vi "视频播放.vi"() -> ()   [LabVIEW 2014]
panel:
  out "Image 2":T1(plugin-control)
  out "Image":T1(plugin-control)
  in  "Image Type":T2 items=["Grayscale (U8)", "Grayscale (I16)", "Grayscale (SGL)", "Complex (CSG)", "RGB (U32)", "HSL (U32)", "RGB (U64)", "Grayscale (U16)"]
  in  "Image Name":string="untitled"
  in  "AVI Path":path
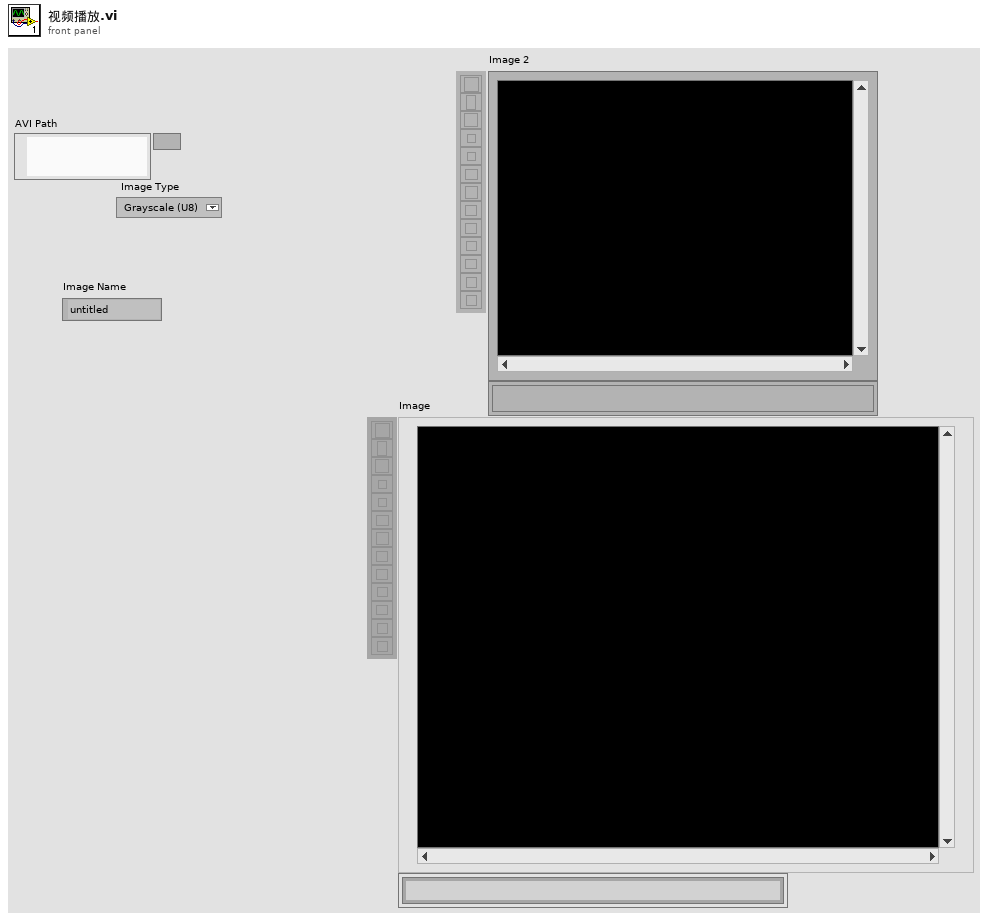
[diagram p1: front panel]
types:
  T1 = typedef "IMAQ Image.ctl" = refnum<image>
  T2 = typedef "Image Type" = u32
  T3 = typedef "AviRefnum.ctl" = refnum<k1>
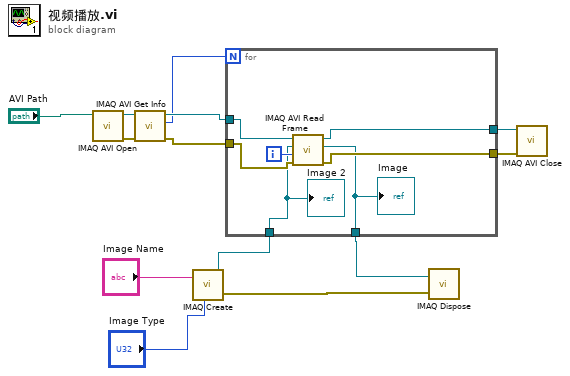
[diagram p0: block diagram]
diagram:
  n1 = call "IMAQ AVI Open"("AVI Path"="AVI Path") -> ("error out"=w10:errorcluster, "Avi Refnum"=w13:T3)  [unwired: 9 in]
  n2 = call "IMAQ AVI Get Info"("error in (no error)"=w10, "Avi Refnum"=w13) -> ("error out"=w9:errorcluster, "Number of Frames"=w1:u32, "Avi Refnum (duplicate)"=w12:T3)  [unwired: 5 in, 2 out]
  n3 = call "IMAQ Create"("Image Name"="Image Name", "Image Type"="Image Type") -> ("New Image"=w6:T1, "error out"=w4:errorcluster)  [unwired: 3 in]
  n4 = for {
    N: w1 -> [_]
    tunnel: w12 -> [w20]
    tunnel: w9 -> [w19]
    tunnel: [w18] -> w8
    tunnel: [w17] -> w7
    tunnel: w6 -> [w15]
    tunnel: [w14] -> w5
    i -> [w16]
    n5 = call "IMAQ AVI Read Frame"("error in (no error)"=w19, "Frame Number"=w16, "Image"=w15, "Avi Refnum"=w20) -> ("error out"=w17:errorcluster, "Image Out"=w14:T1, "Avi Refnum (duplicate)"=w18:T3)  [unwired: 4 in, 1 out]
    "Image" <- w14
    "Image 2" <- w15
  }
  n6 = call "IMAQ Dispose"("Image"=w5, "error in (no error)"=w4) -> ()  [unwired: 4 in, 1 out]
  n7 = call "IMAQ AVI Close"("error in (no error)"=w7, "Avi Refnum"=w8) -> ()  [unwired: 9 in, 1 out]
